vi "Autonomous Independent.vi"   [LabVIEW 2014]
doc: "This VI is called when autonomous begins, and will automatically be terminated when autonomous ends. You can carry out timed or sensor driven robot movement independently without needing to return to the caller."
uses:
  <vilib>/Rock Robotics/Network Tables/SD Read Boolean.vi
panel:
  # "Be sure to right-click and choose Data Operations>>Make Current Value default if you want to save the array values with the VI"
types:
  T1 = typedef "WPI_JoystickDevRef.ctl" = cluster{"Device":T2}
  T2 = typedef "WPI_JoystickDeviceEnum.ctl" = enum16{"USB 0", "USB 1", "USB 2", "USB 3", "USB 4", "USB 5"}
  T3 = typedef "WPI_GyroDevRef.ctl" = cluster{"DevStatus":errorcluster, "Analog Module":T4, "Analog Channel":T5, "Offset":dbl, "Gain (VoltsPerDegree/Second)":dbl}
  T4 = typedef "FPGA_TypedefAnalogModule.ctl" = enum16{"Controller 1"}
  T5 = typedef "FPGA_AIChannel.ctl" = enum8{"AI 0", "AI 1", "AI 2", "AI 3", "AI MXP 0", "AI MXP 1", "AI MXP 2", "AI MXP 3", "Invalid"}
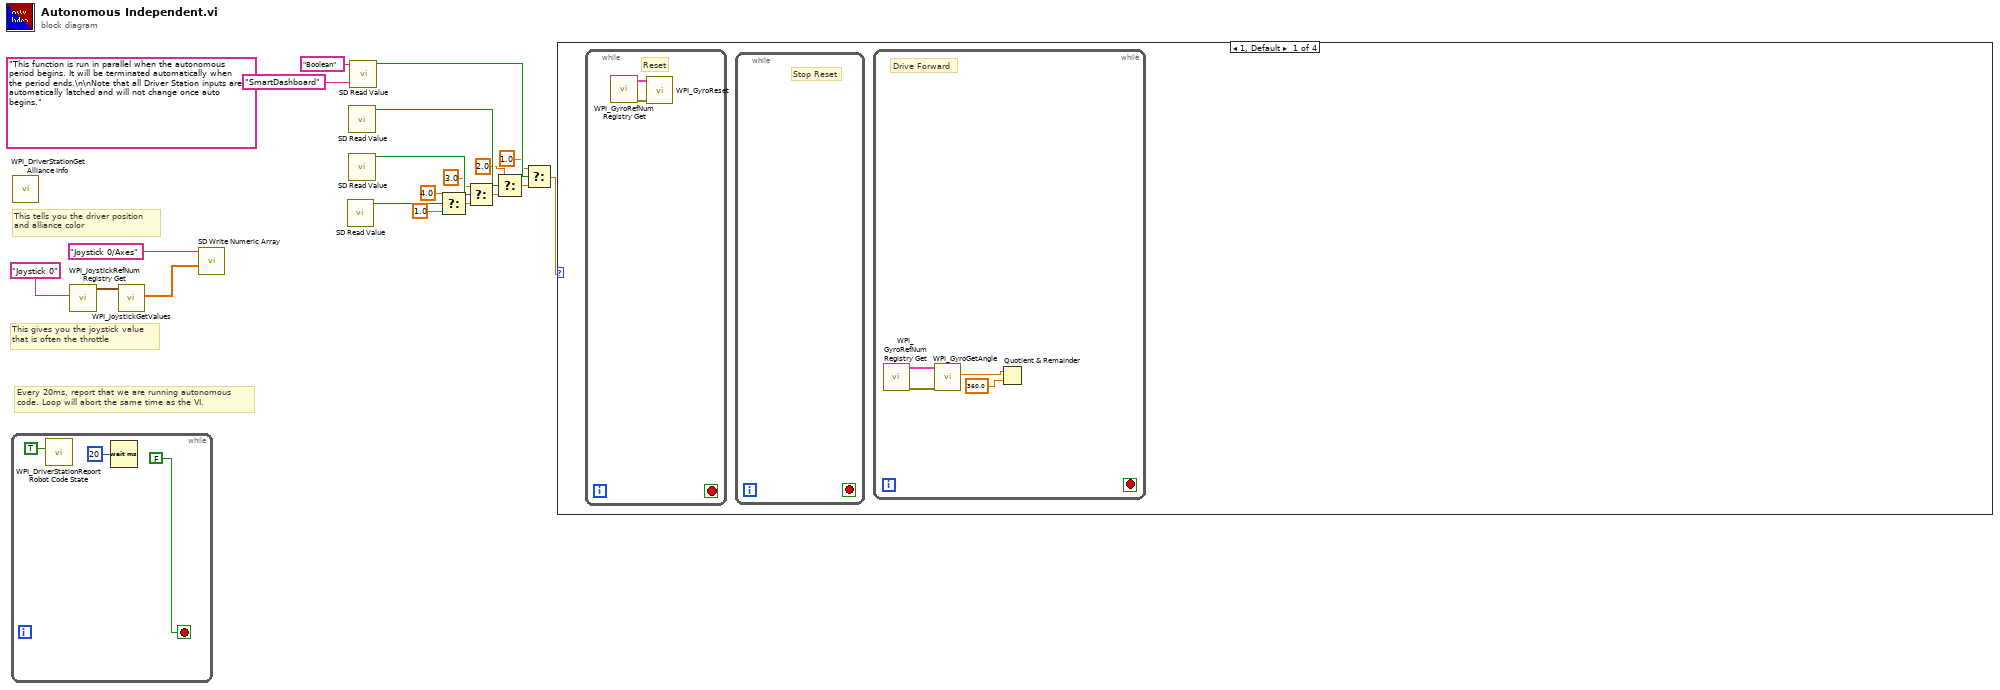
[diagram p0: block diagram]
diagram:
  (unwired) "This function is run in parallel when the autonomous period begins. It will be terminated automatically when the period ends.\n\nNote that all Driver Station inputs are automatically latched and will not change once auto begins."
  # "Every 20ms, report that we are running autonomous\ncode. Loop will abort the same time as the VI."
  # "This gives you the joystick value\nthat is often the throttle"
  # "This tells you the driver position\nand alliance color"
  n1 = while {
    stop <- FALSE stop-if-true
    n2 = call <vilib>:"WPI_DriverStationReport Robot Code State.vi"("Autonomous"=TRUE) -> ()  [unwired: 10 in, 1 out]
    n3 = Wait (ms)(milliseconds to wait=u32 20) -> ()  [unwired: 1 out]
  }
  n4 = call <vilib>:"WPI_DriverStationGet Alliance Info.vi"() -> ()  [unwired: 12 out]
  n5 = call <vilib>:"WPI_JoystickRefNum Registry Get.vi"("refnum name"="Joystick 0") -> ("JoystickDevRef"=w18:T1)  [unwired: 1 in, 9 out]
  n6 = call <vilib>:"WPI_JoystickGetValues.vi"("JoystickDevRef"=w18) -> ("Axes"=w16:dbl[])  [unwired: 6 in, 4 out]
  n7 = call <vilib>:"SD Write Numeric Array.vi"("Numeric Array"=w16, "Name"="Joystick 0/Axes") -> ()  [unwired: 8 in, 2 out]
  n8 = call-poly <vilib>:"SD Read Value.vi"() -> ("Boolean"=w10:bool)  [unwired: 9 in, 2 out]
  n9 = call-poly <vilib>:"SD Read Value.vi"() -> ("Boolean"=w8:bool)  [unwired: 9 in, 2 out]
  n10 = call-poly <vilib>:"SD Read Value.vi"() -> ("Boolean"=w9:bool)  [unwired: 9 in, 2 out]
  n11 = call-poly <vilib>:"SD Read Value.vi"("Table Prefix"="SmartDashboard", "Name"="Boolean") -> ("Boolean"=w7:bool)  [unwired: 7 in, 2 out]
  n12 = Select(t=4.0 ("f"), s=w10, f=1.0) -> (s? t:f=w13:dbl)
  n13 = Select(t=3.0 ("f"), s=w9, f=w13) -> (s? t:f=w12:dbl)
  n14 = Select(t=2.0 ("f"), s=w8, f=w12) -> (s? t:f=w11:dbl)
  n15 = Select(t=1.0 ("f"), s=w7, f=w11) -> (s? t:f=w1:dbl)
  n16 = case shown="1, Default" w1 {
    frame 1, Default {
      n17 = while {
        stop <- _ stop-if-true
        # "Reset"
        n18 = call <vilib>:"WPI_GyroRefNum Registry Get.vi"() -> ("error out"=w27:errorcluster, "GyroDevRef"=w28:T3)  [unwired: 10 in]
        n19 = call <vilib>:"WPI_GyroReset.vi"("error in (no error)"=w27, "GyroDevRef"=w28) -> ()  [unwired: 8 in, 2 out]
      }
      n20 = while {
        stop <- _ stop-if-true
        # "Stop Reset"
      }
      n21 = while {
        stop <- _ stop-if-true
        # "Drive Forward"
        n22 = call <vilib>:"WPI_GyroRefNum Registry Get.vi"() -> ("error out"=w26:errorcluster, "GyroDevRef"=w25:T3)  [unwired: 10 in]
        n23 = call <vilib>:"WPI_GyroGetAngle.vi"("error in (no error)"=w26, "GyroDevRef"=w25) -> ("Angle"=w24:dbl)  [unwired: 6 in, 3 out]
        n24 = Quotient & Remainder(x=w24, y=360.0) -> ()  [unwired: 2 out]
      }
    }
    frame 2 {
    }
    frame 3 {
    }
    frame 4 {
    }
  }
